vi "Load Reference.vi"(8 "error in (no error)":errorcluster, 10 "Reference":refnum<vi>, 11 "SingleStepTestV3 in":refnum<class "SingleStepCODMnV2.lvclass">) -> (0 "error out":errorcluster, 3 "SingleStepTestV3 out":refnum<class "SingleStepCODMnV2.lvclass">)   [LabVIEW 2022 SP3, in "SingleStepCODMnV2.lvlib" / "SingleStepCODMnV2.lvclass"]
doc: "The <b>Load Reference VI</b> is a dynamic dispatch VI that must be overwritten in every QControl Class and must <b>Call Parent Method</b>. This recursively loads the reference of the control to the data space for the Control Class up the inheritance hierarchy (class hierarchy). These references must be loaded in this way to use all of the built-in properties.\n\nThe reference input is the reference type needed for the control but is coerced to Generic. It should be cast back to the correct type before bundling into the class private data. The pre-casted \"Generic\" reference is wired as input to the <b>Call Parent Method</b>.\n<b> </b> <b> </b>\n©2016 Q Software Innovations, LLC (QSI)\nwritten by Quentin Alldredge\nproduced in LabVIEW 2015\n\nsupport@qsoftwareinnovations.com\nwww.qsoftwareinnovations.com\n\nAll rights reserved.\n\nRedistribution and use in source and binary forms, with or without modification, are permitted provided that the following conditions are met:\n\n * Redistributions of source code must retain the above copyright notice, this list of conditions and the following disclaimer.\n * Redistributions in binary form must reproduce the above copyright notice, this list of conditions and the following disclaimer in the documentation and/or other materials provided with the distribution.\n * Neither the name of Q Software Innovations, LLC. nor the names of its contributors may be used to endorse or promote products derived from this software without specific prior written permission.\n\nTHIS SOFTWARE IS PROVIDED BY THE COPYRIGHT HOLDERS AND CONTRIBUTORS \"AS IS\" AND ANY EXPRESS OR IMPLIED WARRANTIES, INCLUDING, BUT NOT LIMITED TO, THE IMPLIED WARRANTIES OF MERCHANTABILITY AND FITNESS FOR A PARTICULAR PURPOSE ARE DISCLAIMED. IN NO EVENT SHALL THE COPYRIGHT OWNER OR CONTRIBUTORS BE LIABLE FOR ANY DIRECT, INDIRECT, INCIDENTAL, SPECIAL, EXEMPLARY, OR CONSEQUENTIAL DAMAGES (INCLUDING, BUT NOT LIMITED TO, PROCUREMENT OF SUBSTITUTE GOODS OR SERVICES; LOSS OF USE, DATA, OR PROFITS; OR BUSINESS INTERRUPTION) HOWEVER CAUSED AND ON ANY THEORY OF LIABILITY, WHETHER IN CONTRACT, STRICT LIABILITY, OR TORT (INCLUDING NEGLIGENCE OR OTHERWISE) ARISING IN ANY WAY OUT OF THE USE OF THIS SOFTWARE, EVEN IF ADVISED OF THE POSSIBILITY OF SUCH DAMAGE."
uses:
  SingleStepCODMnV2.lvclass
  SingleStepCODMnV2.lvclass/SingleStepCODMnV2.ctl
  <vilib>/QSI/QControls/QControl Classes/Cluster/Cluster.lvclass
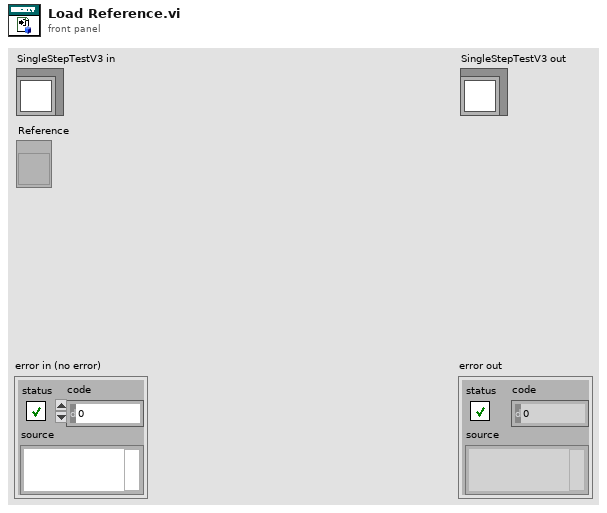
[diagram p1: front panel]
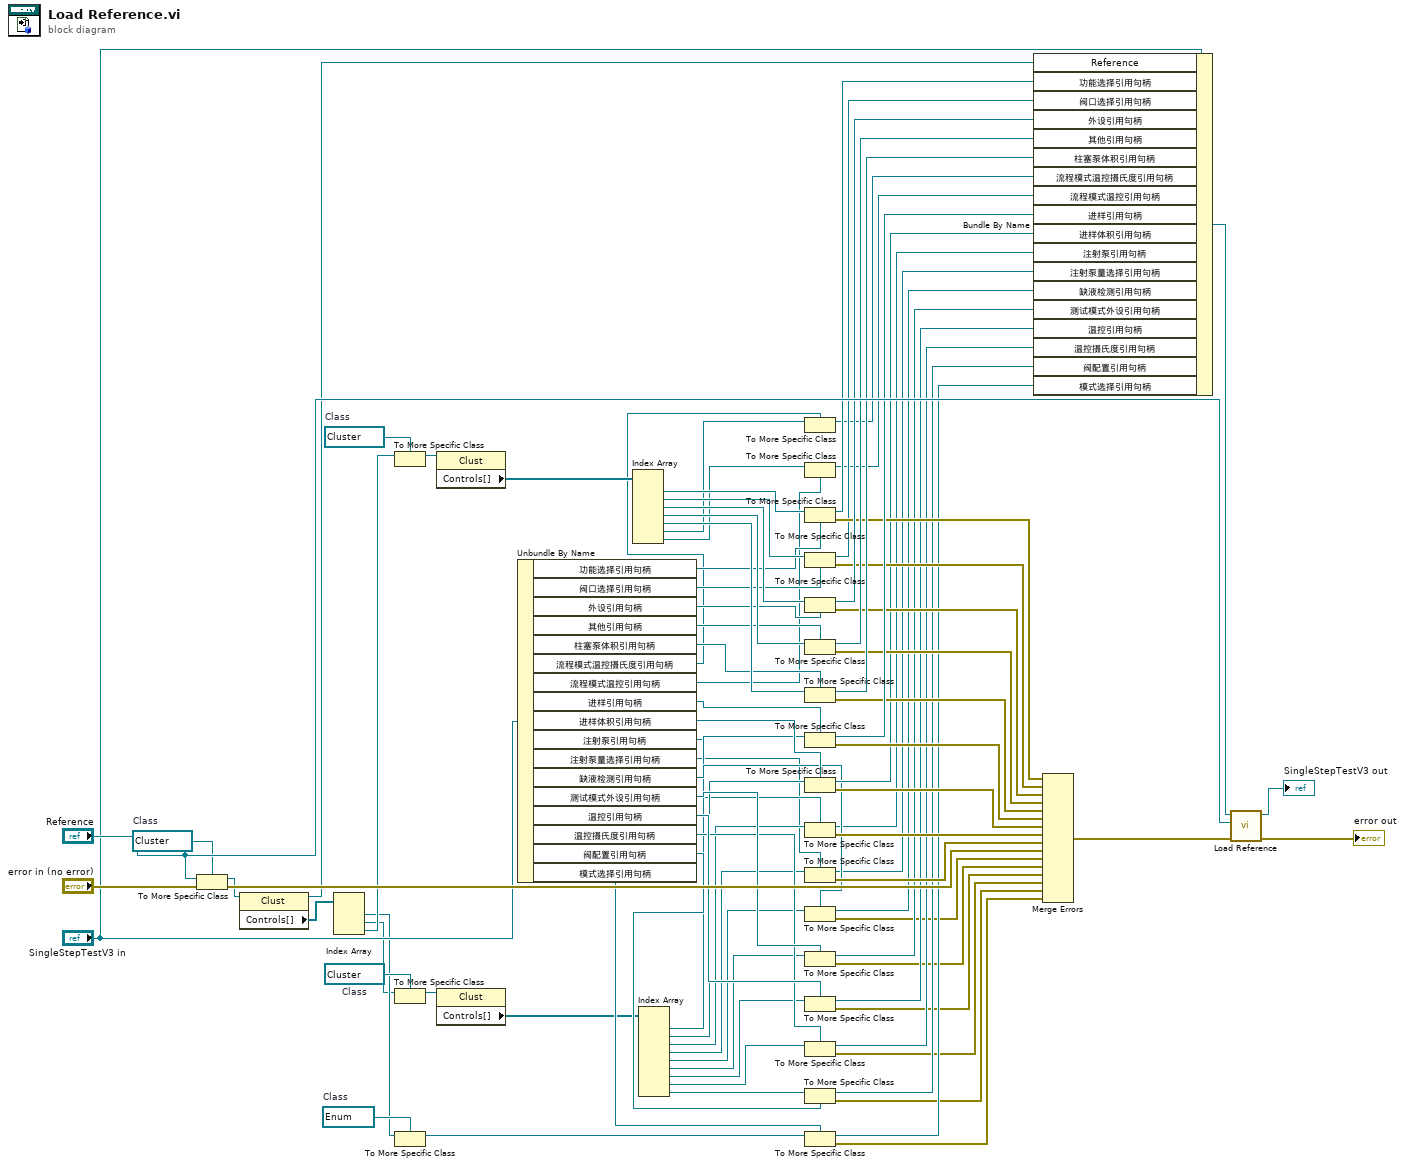
[diagram p0: block diagram]
diagram:
  w18 = refnum<vi> refnum  # Class
  w26 = refnum<vi> refnum  # Class
  w31 = refnum<vi> refnum  # Class
  w86 = refnum<vi> refnum  # Class
  n1 = To More Specific Class(target class=w86, reference="Reference", error in="error in (no error)") -> (specific class reference=w81:refnum<vi>, error out=w88:errorcluster)
  n2 = property class="Clust"(reference=w81) -> (reference out=w33:refnum<vi>, "Controls[]"=w29:refnum<vi>[])  [unwired: 1 in, 1 out]
  n3 = Index Array(array=w29) -> (element #1=w8:refnum<vi>, element #2=w7:refnum<vi>, element #3=w9:refnum<vi>)  [unwired: 3 in]
  n4 = To More Specific Class(target class=w31, reference=w9) -> (specific class reference=w30:refnum<vi>)  [unwired: 1 in, 1 out]
  n5 = To More Specific Class(target class=w26, reference=w7) -> (specific class reference=w27:refnum<vi>)  [unwired: 1 in, 1 out]
  n6 = To More Specific Class(target class=w18, reference=w8) -> (specific class reference=w10:refnum<vi>)  [unwired: 1 in, 1 out]
  n7 = property class="Clust"(reference=w30) -> ("Controls[]"=w28:refnum<vi>[])  [unwired: 1 in, 2 out]
  n8 = property class="Clust"(reference=w27) -> ("Controls[]"=w25:refnum<vi>[])  [unwired: 1 in, 2 out]
  n9 = Unbundle By Name("SingleStepTestV3 in") -> ("功能选择引用句柄"=w58:refnum<vi>, "阀口选择引用句柄"=w57:refnum<vi>, "外设引用句柄"=w56:refnum<vi>, "其他引用句柄"=w55:refnum<vi>, "柱塞泵体积引用句柄"=w54:refnum<vi>, "流程模式温控摄氏度引用句柄"=w6:refnum<vi>, "流程模式温控引用句柄"=w3:refnum<vi>, "进样引用句柄"=w53:refnum<vi>, "进样体积引用句柄"=w52:refnum<vi>, "注射泵引用句柄"=w14:refnum<vi>, "注射泵量选择引用句柄"=w13:refnum<vi>, "缺液检测引用句柄"=w51:refnum<vi>, "测试模式外设引用句柄"=w50:refnum<vi>, "温控引用句柄"=w49:refnum<vi>, "温控摄氏度引用句柄"=w48:refnum<vi>, "阀配置引用句柄"=w47:refnum<vi>, "模式选择引用句柄"=w46:refnum<vi>)
  n10 = Index Array(array=w28) -> (element #1=w32:refnum<vi>, element #2=w80:refnum<vi>, element #3=w79:refnum<vi>, element #4=w77:refnum<vi>, element #5=w73:refnum<vi>, element #6=w5:refnum<vi>, element #7=w2:refnum<vi>)  [unwired: 7 in]
  n11 = Index Array(array=w25) -> (element #1=w15:refnum<vi>, element #2=w16:refnum<vi>, element #3=w17:refnum<vi>, element #4=w24:refnum<vi>, element #5=w23:refnum<vi>, element #6=w22:refnum<vi>, element #7=w21:refnum<vi>, element #8=w20:refnum<vi>, element #9=w19:refnum<vi>)  [unwired: 9 in]
  n12 = To More Specific Class(target class=w6, reference=w5) -> (specific class reference=w4:refnum<vi>)  [unwired: 1 in, 1 out]
  n13 = To More Specific Class(target class=w3, reference=w2) -> (specific class reference=w1:refnum<vi>)  [unwired: 1 in, 1 out]
  n14 = To More Specific Class(target class=w58, reference=w32) -> (specific class reference=w62:refnum<vi>, error out=w63:errorcluster)  [unwired: 1 in]
  n15 = To More Specific Class(target class=w57, reference=w80) -> (specific class reference=w61:refnum<vi>, error out=w64:errorcluster)  [unwired: 1 in]
  n16 = To More Specific Class(target class=w56, reference=w79) -> (specific class reference=w78:refnum<vi>, error out=w65:errorcluster)  [unwired: 1 in]
  n17 = To More Specific Class(target class=w55, reference=w77) -> (specific class reference=w76:refnum<vi>, error out=w66:errorcluster)  [unwired: 1 in]
  n18 = To More Specific Class(target class=w54, reference=w73) -> (specific class reference=w75:refnum<vi>, error out=w67:errorcluster)  [unwired: 1 in]
  n19 = To More Specific Class(target class=w53, reference=w15) -> (specific class reference=w74:refnum<vi>, error out=w68:errorcluster)  [unwired: 1 in]
  n20 = To More Specific Class(target class=w52, reference=w16) -> (specific class reference=w60:refnum<vi>, error out=w69:errorcluster)  [unwired: 1 in]
  n21 = To More Specific Class(target class=w14, reference=w17) -> (specific class reference=w12:refnum<vi>, error out=w70:errorcluster)  [unwired: 1 in]
  n22 = To More Specific Class(target class=w13, reference=w24) -> (specific class reference=w11:refnum<vi>, error out=w71:errorcluster)  [unwired: 1 in]
  n23 = To More Specific Class(target class=w51, reference=w23) -> (specific class reference=w45:refnum<vi>, error out=w39:errorcluster)  [unwired: 1 in]
  n24 = To More Specific Class(target class=w50, reference=w22) -> (specific class reference=w43:refnum<vi>, error out=w38:errorcluster)  [unwired: 1 in]
  n25 = To More Specific Class(target class=w49, reference=w21) -> (specific class reference=w44:refnum<vi>, error out=w37:errorcluster)  [unwired: 1 in]
  n26 = To More Specific Class(target class=w48, reference=w20) -> (specific class reference=w42:refnum<vi>, error out=w36:errorcluster)  [unwired: 1 in]
  n27 = To More Specific Class(target class=w47, reference=w19) -> (specific class reference=w41:refnum<vi>, error out=w35:errorcluster)  [unwired: 1 in]
  n28 = To More Specific Class(target class=w46, reference=w10) -> (specific class reference=w40:refnum<vi>, error out=w34:errorcluster)  [unwired: 1 in]
  n29 = Bundle By Name(cluster="SingleStepTestV3 in", "Reference"=w33, "功能选择引用句柄"=w62, "阀口选择引用句柄"=w61, "外设引用句柄"=w78, "其他引用句柄"=w76, "柱塞泵体积引用句柄"=w75, "流程模式温控摄氏度引用句柄"=w4, "流程模式温控引用句柄"=w1, "进样引用句柄"=w74, "进样体积引用句柄"=w60, "注射泵引用句柄"=w12, "注射泵量选择引用句柄"=w11, "缺液检测引用句柄"=w45, "测试模式外设引用句柄"=w43, "温控引用句柄"=w44, "温控摄氏度引用句柄"=w42, "阀配置引用句柄"=w41, "模式选择引用句柄"=w40) -> (w85:refnum<class "SingleStepCODMnV2.lvclass">)
  n30 = Merge Errors(w63, w64, w65, w66, w67, w68, w69, w70, w71, w88, w39, w38, w37, w36, w35, w34) -> (w72:errorcluster)
  n31 = call-parent "Load Reference.vi"("error in (no error)"=w72, "Reference"="Reference", "Cluster in"=w85) -> ("error out"=→"error out":errorcluster, "Cluster out"=→"SingleStepTestV3 out":refnum<class "SingleStepCODMnV2.lvclass">)  [unwired: 7 in]
